vi "SaveFile.vi"(8 "error in (no error)":errorcluster, 9 "Data":string, 10 "Filename":string, 11 "TCP_Client in":refnum<class "TCP_Client.lvclass">) -> (0 "error out":errorcluster, 3 "TCP_Client out":refnum<class "TCP_Client.lvclass">)   [LabVIEW 2023, in "TCP_Client.lvlib" / "TCP_Client.lvclass"]
uses:
  TCP_Client.lvclass
  TCP_Client.lvclass/TCP_Client.ctl
  <vilib>/Utility/error.llb/DialogType.ctl
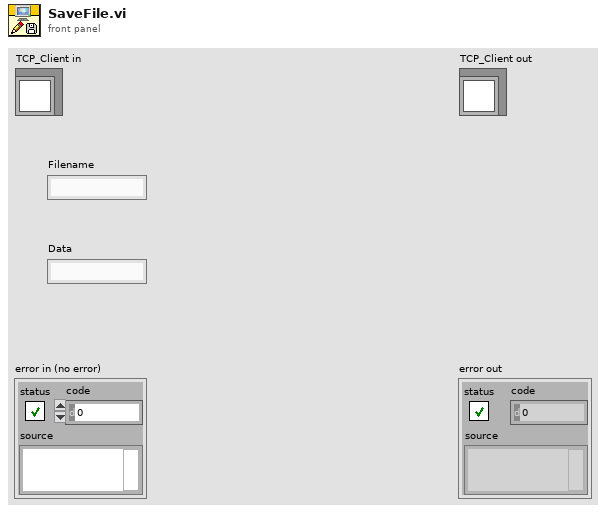
[diagram p1: front panel]
types:
  T1 = enum16{"open", "replace", "create", "open or create", "replace or create", "replace or create with confirmation"}
  T2 = typedef "DialogType.ctl" = u16
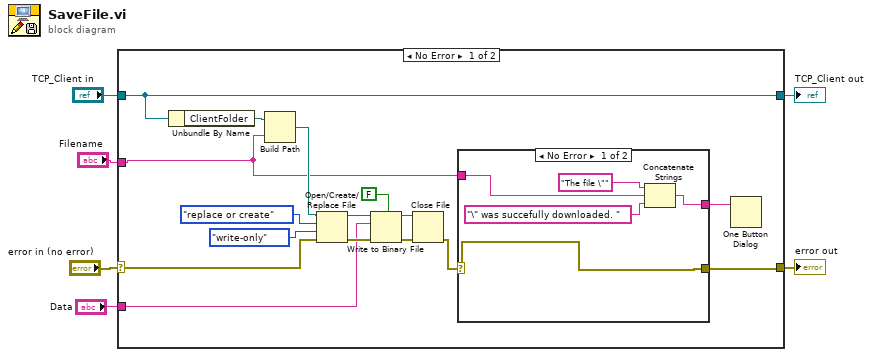
[diagram p0: block diagram]
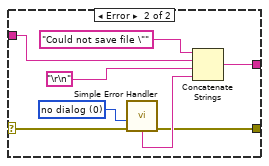
[diagram p2: hidden frame]
diagram:
  n1 = case shown="No Error" "error in (no error)" {
    selector: "error in (no error)" -> [w10 w37]
    tunnel: [w7 w37] -> w5
    tunnel: [w13 w36] -> w3
    tunnel: "TCP_Client in" -> [w13 w36]
    tunnel: "Filename" -> [w11 _]
    tunnel: "Data" -> [w9 _]
    frame No Error {
      n2 = Unbundle By Name(w13) -> ("ClientFolder"=w12:path)
      n3 = Build Path(base path=w12, name or relative path=w11) -> (appended path=w22:path)
      n4 = Open/Create/Replace File(file path (use dialog)=w22, error in=w10, operation (0:open)=T1."replace or create", access (0:read/write)=enum16{"read/write", "read-only", "write-only"}."write-only") -> (refnum out=w19:refnum<file>, error out=w18:errorcluster)  [unwired: 2 in, 1 out]
      n5 = Write to Binary File(file (use dialog)=w19, data=w9, error in=w18, 5:FALSE ("prepend array or string size? (T)")) -> (refnum out=w16:refnum<file>, error out=w17:errorcluster)  [unwired: 2 in, 1 out]
      n6 = Close File(refnum=w16, error in=w17) -> (error out=w14:errorcluster)  [unwired: 1 out]
      n7 = case shown="No Error" w14 {
        selector: w14 -> [w23 w32]
        tunnel: w11 -> [w26 w34]
        tunnel: [w23 w29] -> w7
        tunnel: [w24 w28] -> w8
        frame No Error {
          n8 = Concatenate Strings("The file \"", w26, "\" was succefully downloaded. " ("string")) -> (w24:string)
        }
        frame Error {
          w30 = T2 0 items=["no dialog", "OK message", "continue or stop message", "OK message + warnings", "continue/stop + warnings"] ("type of dialog (OK msg:1)")
          n9 = call <vilib>:"Simple Error Handler.vi"("type of dialog (OK msg:1)"=w30, "error in (no error)"=w32) -> ("error out"=w29:errorcluster, "message"=w31:string)  [unwired: 3 in, 3 out]
          n10 = Concatenate Strings("Could not save file \"", w34, "\r\n", w31) -> (w28:string)
        }
      }
      n11 = One Button Dialog(message=w8) -> ()  [unwired: 1 in, 1 out]
    }
    frame Error {
    }
  }
  "error out" <- w5
  "TCP_Client out" <- w3
